vi "Fetch Multi Eval Meas Trace IQ Constellation Results.vi"(8 "error in (no error)":errorcluster, 9 "Window Position (Low)":i32(ring) items=["Low", "High"], 10 "Instance (1)":T1=1, 11 "VISA resource name":refnum<visa-resource-name>) -> (0 "error out":errorcluster, 1 "Trace IQ Constellation Results":cluster{"I Phase":dbl, "Q Phase":dbl}[](array[cluster]) {"Q Phase" format="%^.3e"; "I Phase" format="%^.3e"}, 2 "Reliability":i32, 3 "VISA resource name out":refnum<visa-resource-name>)   [LabVIEW 2015, in "Rohde&Schwarz CMXP NR FR2 Measurement.lvlib"]
doc: "Returns the results in the I/Q constellation diagram for low and high EVM window position.\n\nAttributes:\nRSCMXPNRFR2M_ATTR_FETCH_MULTI_EVAL_MEASUREMENT_TRACE_IQ_HIGH_RESULTS\nRSCMXPNRFR2M_ATTR_FETCH_MULTI_EVAL_MEASUREMENT_TRACE_IQ_LOW_RESULTS\n\nRemote-control commands:\nFETCh:NRMMw:MEAS<i>:MEValuation:TRACe:IQ:HIGH?\nFETCh:NRMMw:MEAS<i>:MEValuation:TRACe:IQ:LOW?"
uses:
  <instrlib>/Rohde&Schwarz CMXP NR FR2 Measurement/Rohde&Schwarz CMXP NR FR2 Measurement.lvlib
  <instrlib>/Rohde&Schwarz CMXP NR FR2 Measurement/Private/_Instance.ctl
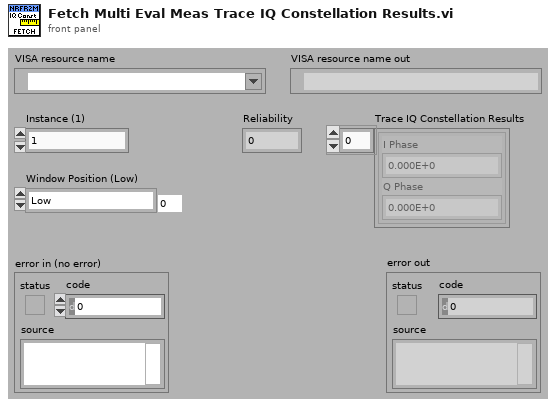
[diagram p1: front panel]
types:
  T1 = typedef "Rohde&Schwarz CMXP NR FR2 Measurement.lvlib/_Instance.ctl" = i32
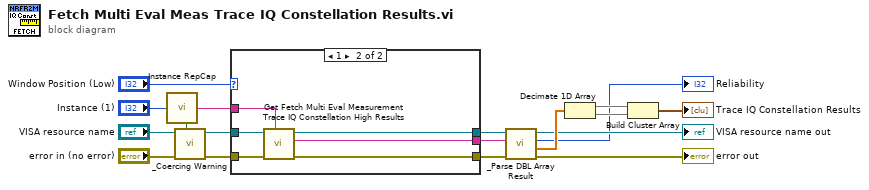
[diagram p0: block diagram]
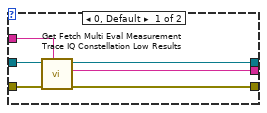
[diagram p2: hidden frame]
diagram:
  n1 = call <instrlib>:"Instance RepCap.vi"("Instance In"="Instance (1)") -> ("In Range?"=w3:bool, "RepCap Identifier Out"=w18:string)  [unwired: 1 in]
  n2 = call <instrlib>:"_Coercing Warning.vi"("In Range?"=w3, "error in (no error)"="error in (no error)", "VISA resource name"="VISA resource name") -> ("error out"=w4:errorcluster, "VISA resource name out"=w5:refnum<visa-resource-name>)  [unwired: 7 in]
  n3 = case shown="1" "Window Position (Low)" {
    tunnel: w4 -> [w24 w30]
    tunnel: w5 -> [w23 w29]
    tunnel: w18 -> [w22 w28]
    tunnel: [w21 w27] -> w14
    tunnel: [w20 w26] -> w13
    tunnel: [w19 w25] -> w12
    frame 0, Default {
      n4 = call "Get Fetch Multi Eval Measurement Trace IQ Constellation Low Results"("Repeated Capabilities"=w22, "error in (no error)"=w24, "instrument handle"=w23) -> ("error out"=w21:errorcluster, "Fetch Multi Eval Measurement Trace IQ Constellation Low Results"=w19:string, "instrument handle out"=w20:refnum<visa-resource-name>)  [unwired: 6 in]
    }
    frame 1 {
      n5 = call "Get Fetch Multi Eval Measurement Trace IQ Constellation High Results"("Repeated Capabilities"=w28, "error in (no error)"=w30, "instrument handle"=w29) -> ("error out"=w27:errorcluster, "Fetch Multi Eval Measurement Trace IQ Constellation High Results"=w25:string, "instrument handle out"=w26:refnum<visa-resource-name>)  [unwired: 6 in]
    }
  }
  n6 = call <instrlib>:"_Parse DBL Array Result.vi"("error in (no error)"=w14, "Input String"=w12, "VISA resource name"=w13) -> ("error out"=→"error out":errorcluster, "Results"=w17:dbl[], "Reliability"=→"Reliability":i32, "VISA resource name out"=→"VISA resource name out":refnum<visa-resource-name>)  [unwired: 5 in]
  n7 = Decimate 1D Array(w17) -> (w16:dbl[], w15:dbl[])
  n8 = Build Cluster Array ("Index & Bundle Cluster Array")(w16, w15) -> (→"Trace IQ Constellation Results":cluster{"Element":dbl, "Element":dbl}[])
